vi "score sorter.vi"(3 "random score":dbl[](array[numeric])) -> (0 "Sorted Cluster":T1)   [LabVIEW 2014]
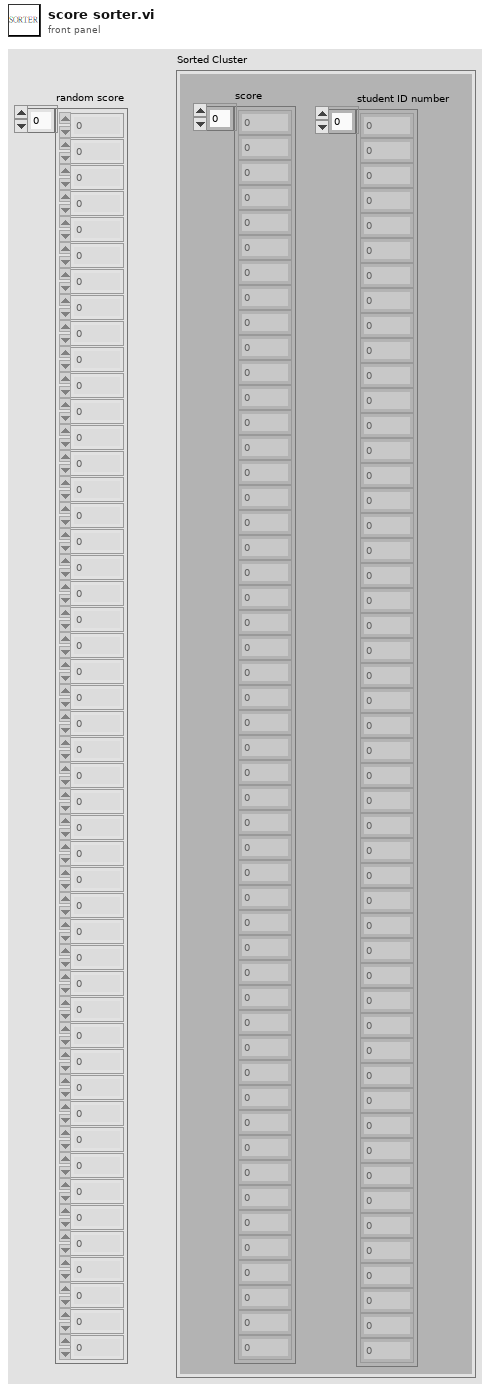
[diagram p1: front panel]
types:
  T1 = cluster{"student ID number":dbl[], "score":dbl[]}
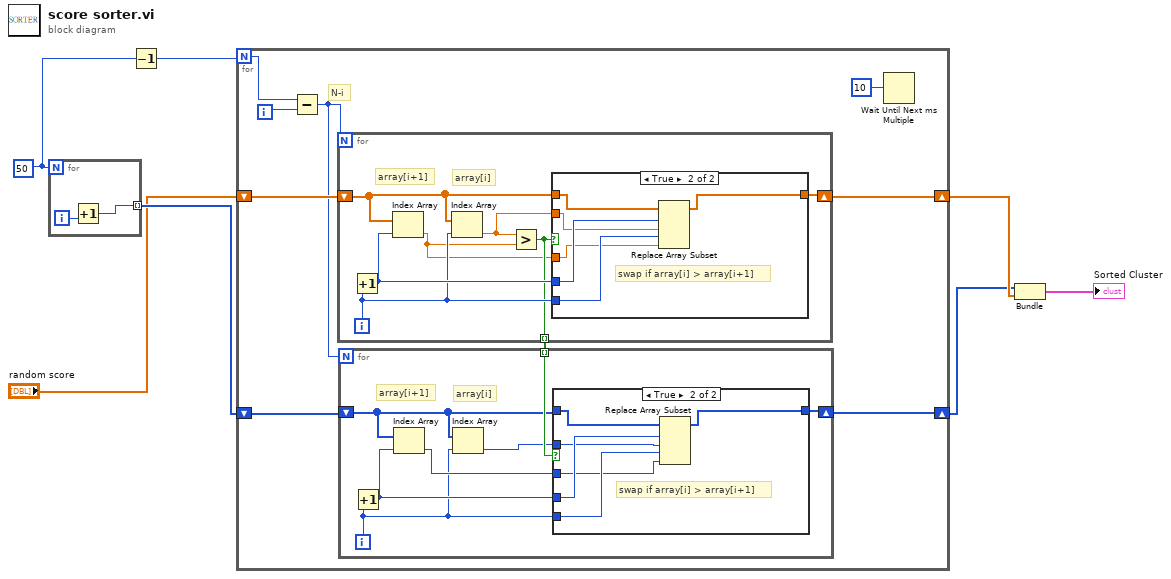
[diagram p0: block diagram]
diagram:
  w7 = 50
  n1 = for {
    N: w7 -> [_]
    tunnel: [w8] -> w4 mode=indexing
    i -> [w9]
    n2 = Increment(x=w9) -> (x+1=w8:i32)
  }
  n3 = Decrement(x=w7) -> (x-1=w2:i32)
  n4 = for {
    N: w2 -> [w18]
    shift-right: [w15] -> w6
    shift-left: "random score" -> [w16]
    shift-right: [w10] -> w5
    shift-left: w4 -> [w11]
    i -> [w17]
    # "N-i"
    n5 = Subtract(x=w18, y=w17) -> (x-y=w12:i32)
    n6 = for {
      N: w12 -> [_]
      shift-right: [w38] -> w15
      shift-left: w16 -> [w39]
      tunnel: [w34] -> w13 mode=indexing
      i -> [w36]
      # "array[i]"
      # "array[i+1]"
      n7 = Increment(x=w36) -> (x+1=w37:i32)
      n8 = Index Array(array=w39, index=w37) -> (element=w33:dbl)
      n9 = Index Array(array=w39, index=w36) -> (element=w35:dbl)
      n10 = Greater?(x=w35, y=w33) -> (0:w34:bool)
      n11 = case shown="True" w34 {
        tunnel: w39 -> [w40 w43]
        tunnel: [w40 w42] -> w38
        tunnel: w36 -> [_ w45]
        tunnel: w37 -> [_ w46]
        tunnel: w35 -> [_ w44]
        tunnel: w33 -> [_ w41]
        frame False {
        }
        frame True {
          # "swap if array[i] > array[i+1]"
          n12 = Replace Array Subset(array=w43, new element #1=w44, index #1=w46, new element #2=w41, index #2=w45) -> (w42:dbl[])
        }
      }
    }
    n13 = for {
      N: w12 -> [_]
      shift-right: [w25] -> w10
      shift-left: w11 -> [w22]
      tunnel: w13 -> [w23] mode=indexing
      i -> [w19]
      # "array[i]"
      # "array[i+1]"
      n14 = Increment(x=w19) -> (x+1=w24:i32)
      n15 = Index Array(array=w22, index=w24) -> (element=w21:i32)
      n16 = Index Array(array=w22, index=w19) -> (element=w20:i32)
      n17 = case shown="True" w23 {
        tunnel: w22 -> [w26 w27]
        tunnel: [w26 w30] -> w25
        tunnel: w19 -> [_ w31]
        tunnel: w24 -> [_ w32]
        tunnel: w21 -> [_ w29]
        tunnel: w20 -> [_ w28]
        frame False {
        }
        frame True {
          # "swap if array[i] > array[i+1]"
          n18 = Replace Array Subset(array=w27, new element #1=w28, index #1=w32, new element #2=w29, index #2=w31) -> (w30:i32[])
        }
      }
    }
    n19 = Wait Until Next ms Multiple(millisecond multiple=10) -> ()  [unwired: 1 out]
  }
  n20 = Bundle(w5, "random score"=w6) -> (→"Sorted Cluster":cluster{i32[], "random score":dbl[]})  [unwired: 1 in]
